vi "Raspberry Pi Compatible Compiler for LabVIEW.vi"() -> ()   [LabVIEW 2014, in "Raspberry Pi Compatible Compiler for LabVIEW.lvlib"]
uses:
  Raspberry Pi Compatible Compiler for LabVIEW.lvlib
  Custom Controls/CompileType.ctl
  RasPi_Services/Download/RuntimeVersion.ctl
  Custom Controls/Local Setup Parameters.ctl
  <vilib>/Platform/browser.llb/Open URL in Default Browser (string).vi
  RasPi_Services/Autodetect/Autodetect.lvlib
  RasPi_Services/Downloader/Downloader.lvclass
  Messaging/SimpleMessaging.lvlib
  RasPi_Services/Download/RasPiDownloader.lvlib
panel:
  in  "exit":bool
  in  "state variables":T2
  in  "Watermark":enum32{"Page 1", "Page 2"}(tab)
  in  "Compile Locally":bool
  out "Animated Image":i16(ring) caption="Ring 2"
  in  "Compilation Type":T3
  in  "Verify Connectivity":bool
  in  "Delete IP":bool
  in  "Edit IP":bool
  in  "Add Ip":bool
  in  "IP List":i32(listbox)
  in  "Blocker":string caption="Status"
  in  "Status":string
  out "Running":bool
  out "VIPath":path caption="Deploy .vi"
  out "StopStat":bool
  in  "FP":bool
  in  "Download":bool
  in  "Help":bool
  in  "Open":bool
  out "Busy":u16(ring)=12
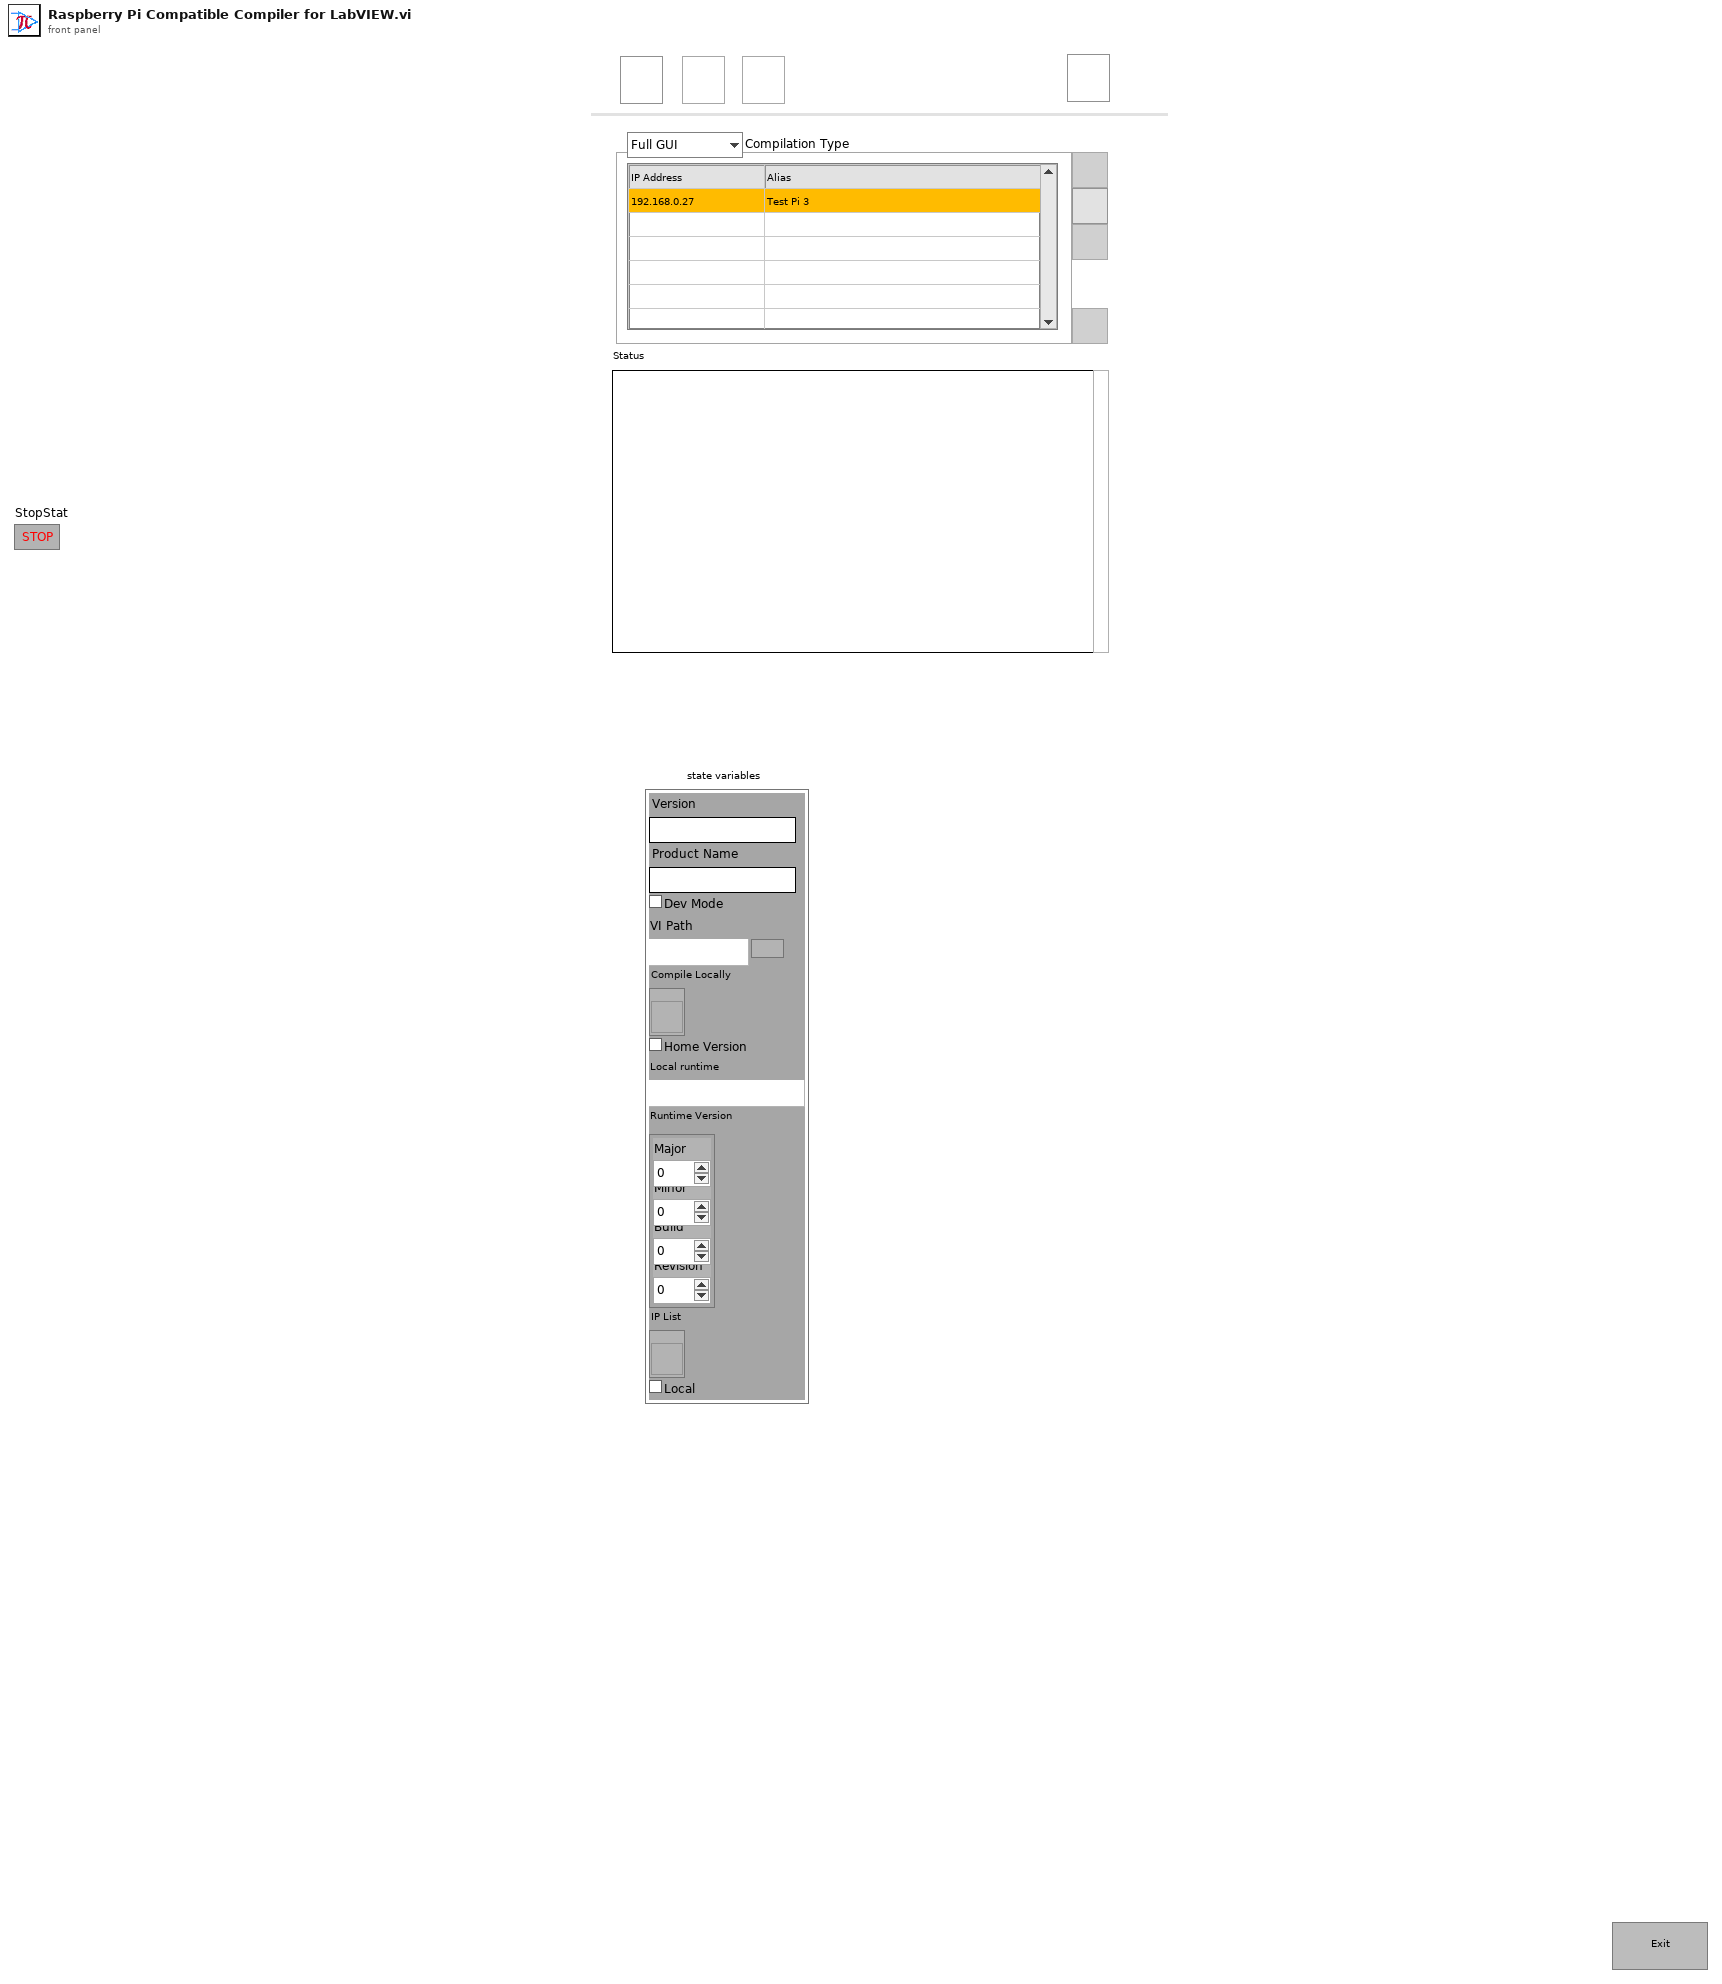
[diagram p1: front panel]
types:
  T1 = typedef "Raspberry Pi Compatible Compiler for LabVIEW.lvlib/RasPiDownloader.lvlib/RuntimeVersion.ctl" = cluster{"Major":i32, "Minor":i32, "Build":i32, "Revision":i32}
  T2 = cluster{"Version":string, "Product Name":string, "Dev Mode":bool, "VI Path":path, "Compile Locally":refnum<vi>, "Home Version":bool, "Local runtime":path, "Runtime Version":T1, "IP List":refnum<vi>, "Local":bool}
  T3 = typedef "Raspberry Pi Compatible Compiler for LabVIEW.lvlib/CompileType.ctl" = enum16{"Full GUI", "Console App"}
  T4 = typedef "Raspberry Pi Compatible Compiler for LabVIEW.lvlib/SimpleMessaging.lvlib/MessageQueueTD.ctl" = refnum<queue>
  T5 = enum8{"Enabled", "Disabled", "Disabled and Grayed Out"}
  T6 = typedef "Raspberry Pi Compatible Compiler for LabVIEW.lvlib/Local Setup Parameters.ctl" = enum16{"Add Last VI", "Read Last VI", "Add Board IP", "Remove Board IP", "Read All Board IP", "Add Runtime Version", "Read Runtime Version", "Add Package Version", "Read Package Version", "Add VIPCheck Time", "Read VIPCheck Time"}
  T7 = enum16{"Add IP", "Delete IP", "Get IP", "Edit IP"}
  T8 = typedef "Raspberry Pi Compatible Compiler for LabVIEW.lvlib/Autodetect.lvlib/UDP_Response_TD.ctl" = cluster{"IP address":string, "Port":u16, "response":string}
  T9 = typedef "Raspberry Pi Compatible Compiler for LabVIEW.lvlib/Autodetect.lvlib/UDP_HostinfoTD.ctl" = cluster{"hostname":string, "version":string}
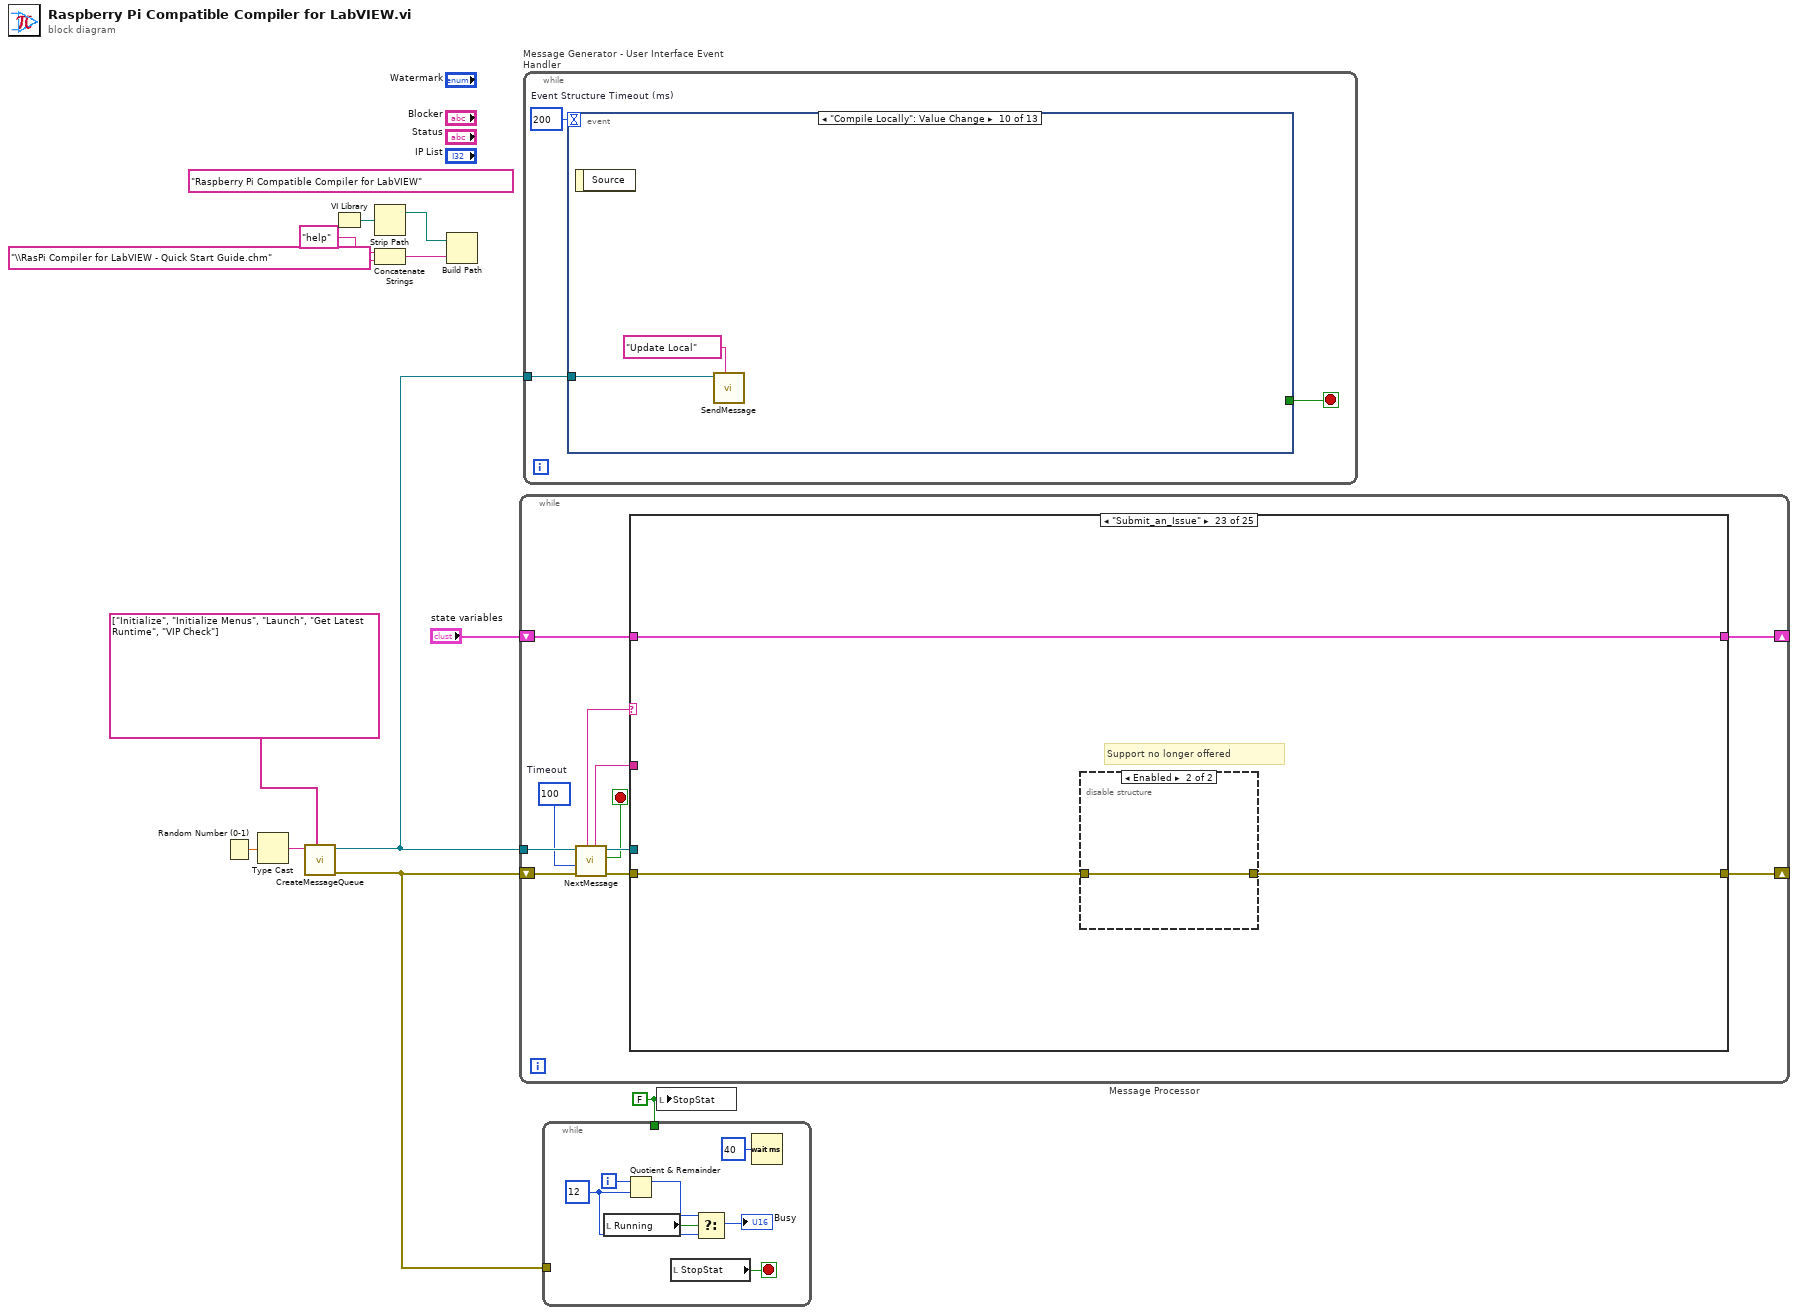
[diagram p0: block diagram]
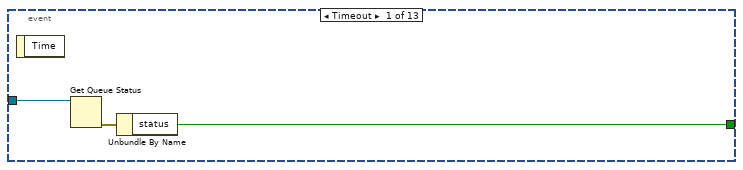
[diagram p2: hidden frame]
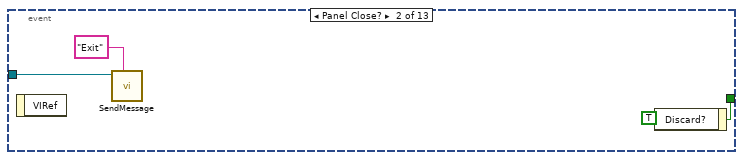
[diagram p3: hidden frame]
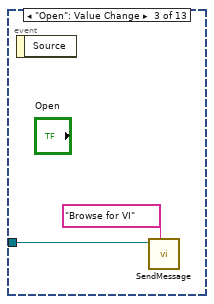
[diagram p4: hidden frame]
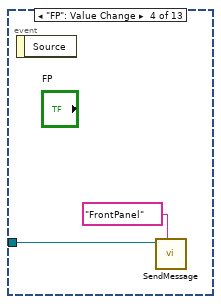
[diagram p5: hidden frame]
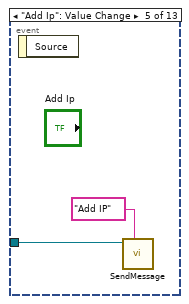
[diagram p6: hidden frame]
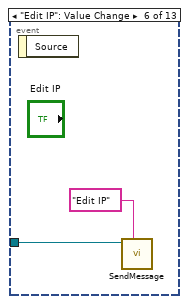
[diagram p7: hidden frame]
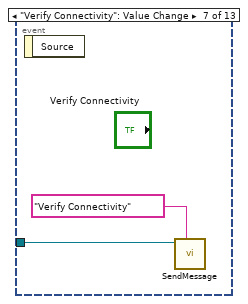
[diagram p8: hidden frame]
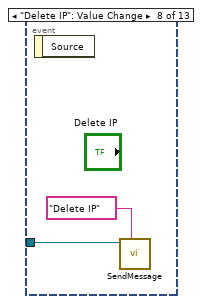
[diagram p9: hidden frame]
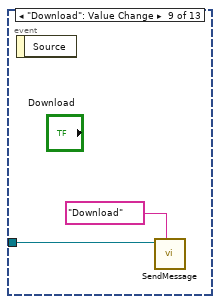
[diagram p10: hidden frame]
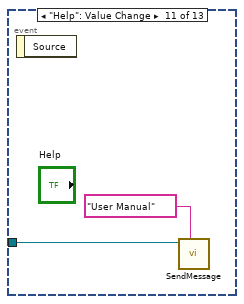
[diagram p11: hidden frame]
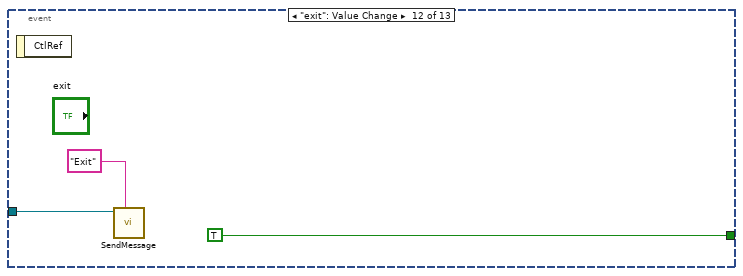
[diagram p12: hidden frame]
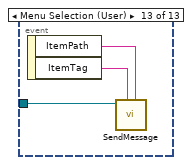
[diagram p13: hidden frame]
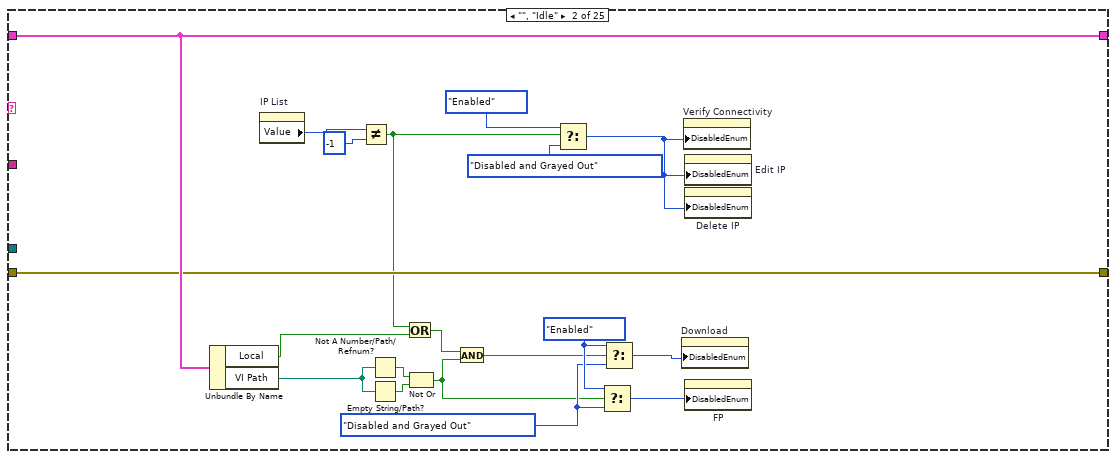
[diagram p15: hidden frame]
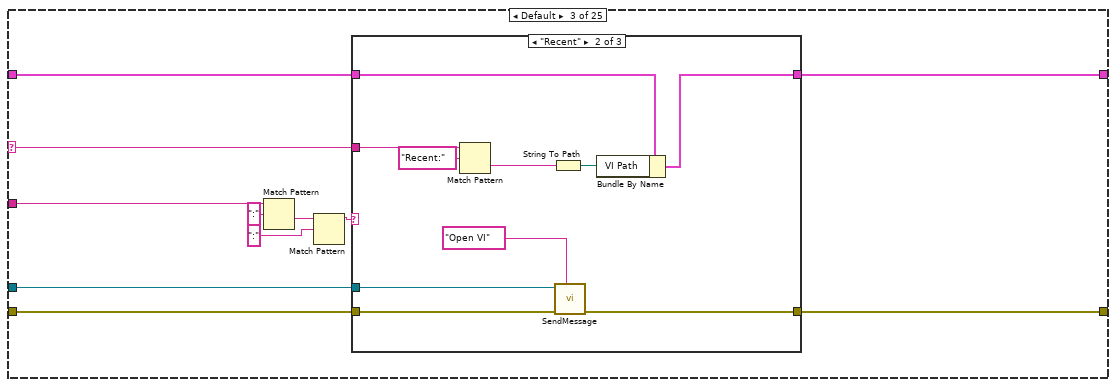
[diagram p16: hidden frame]
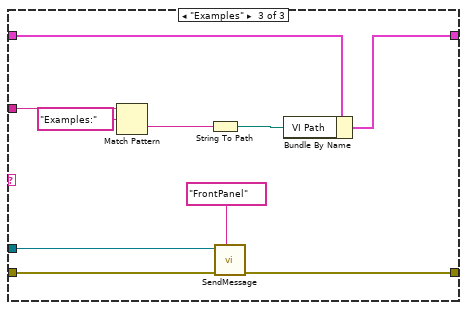
[diagram p18: hidden frame]
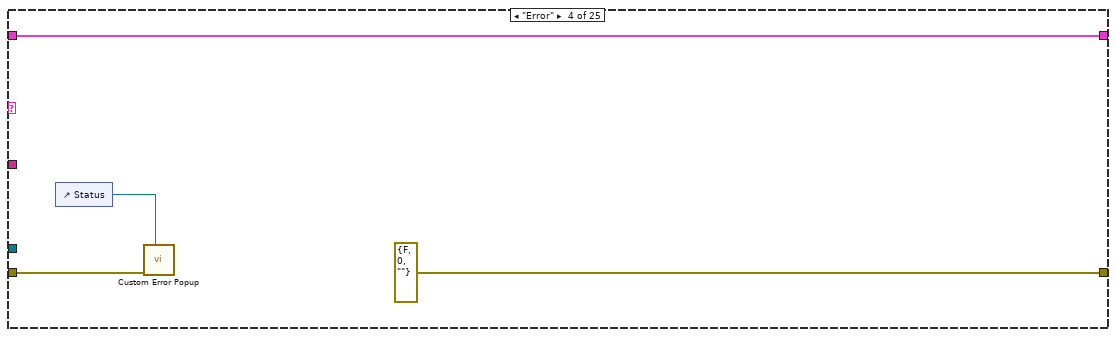
[diagram p19: hidden frame]
diagram:
  w7 = FALSE ("StopStat")
  (unwired) "Raspberry Pi Compatible Compiler for LabVIEW" ("menu tag")
  n1 = Random Number (0-1)() -> (number: 0 to 1=w2:dbl)
  n2 = Type Cast(x=w2) -> (*(type *) &x=w3:string)  [unwired: 1 in]
  n3 = call "CreateMessageQueue.vi"("initial message names"=string[] ["Initialize", "Initialize Menus", "Launch", "Get Latest Runtime", "VIP Check"], "message queue name"=w3) -> ("error out"=w1:errorcluster, "message queue out"=w5:T4)  [unwired: 5 in, 1 out]
  n4 = VI Library() -> (path=w10:path)
  n5 = Strip Path(path=w10) -> (stripped path=w11:path)  [unwired: 1 out]
  n6 = Concatenate Strings("help" ("name or relative path"), "\\RasPi Compiler for LabVIEW - Quick Start Guide.chm" ("name or relative path")) -> (w9:string)
  n7 = Build Path(base path=w11, name or relative path=w9) -> ()  [unwired: 1 out]
  n8 = while "Message Processor" {
    shift-left: w1 -> [w18]
    shift-right: [w21] -> _
    tunnel: w5 -> [w19]
    shift-left: "state variables" -> [w23]
    shift-right: [w22] -> _
    stop <- w13 stop-if-true
    w16 = 100  # Timeout
    n9 = call "NextMessage.vi"("error in"=w18, "timeout in ms (-1)"=w16, "message queue in"=w19) -> ("error out"=w17:errorcluster, "exit"=w13:bool, "message queue out"=w20:T4, "Value"=w14:string, "Name"=w15:string)  [unwired: 1 in, 1 out]
    n10 = case shown="\"Submit_an_Issue\"" w15 {
      selector: w15 -> [_ _ w51 _ _ _ _ _ _ _ _ _ _ _ _ _ _ _ _ _ _ _ _ _ _]
      tunnel: [w25 w35 w46 w81 w83 w111 w123 w140 w188 w224 w238 w246 w248 w249 w284 w317 w330 w335 w348 w368 w403 w415 w418 w428 w433] -> w22
      tunnel: w23 -> [w25 w35 w47 w81 w83 w113 w123 w141 w189 w226 w239 w246 w248 w250 w284 w317 w330 w335 w348 w368 w403 w415 w418 w428 w436]
      tunnel: w20 -> [_ _ w48 _ _ _ _ _ w182 _ _ w244 _ w251 _ _ _ _ _ _ _ _ _ w425 _]
      tunnel: w17 -> [w24 w34 w50 w79 w82 w94 w126 w143 w191 w228 w237 w245 w247 w253 w287 w318 w333 w337 w351 w370 w407 w413 w417 w427 w437]
      tunnel: [w24 w34 w49 errorcluster {"status"=FALSE, "code"=0, "source"=""} ("error out") w82 w87 w125 _ w181 w221 w237 w240 w247 w252 w286 w319 w332 w336 w349 w369 w405 w412 w416 w426 w430] -> w21
      tunnel: w14 -> [_ _ w45 _ _ _ _ _ w177 _ _ _ _ _ _ _ _ _ _ _ _ _ _ _ _]
      frame "---------- Framework Operations ----------" {
      }
      frame "", "Idle" {
        w33 = T5."Disabled and Grayed Out" ("Disabled")
        w38 = T5."Enabled" ("Disabled")
        n11 = Unbundle By Name(w35) -> ("Local"=w26:bool, "VI Path"=w30:path)
        n12 = property on="IP List" class="MCListbox (strict)"() -> ("Value"=w44:i32)  [unwired: 2 in, 2 out]
        n13 = Not Equal?(x=w44, y=-1) -> (x != y?=w31:bool)
        n14 = Not A Number/Path/Refnum?(number/path/refnum=w30) -> (NaN/Path/Refnum?=w28:bool)
        n15 = Empty String/Path?(string/path=w30) -> (empty?=w29:bool)
        n16 = Or(x=w31, y=w26) -> (x .or. y?=w32:bool)
        n17 = Not Or(1:w29, 2:w28) -> (0:w27:bool)
        n18 = And(x=w32, y=w27) -> (x .and. y?=w36:bool)
        n19 = Select(t=T5."Enabled", s=w31, f=T5."Disabled and Grayed Out" ("Disabled")) -> (s? t:f=w40:T5)
        n20 = Select(t=w38, s=w27, f=w33) -> (s? t:f=w37:T5)
        n21 = Select(t=w38, s=w36, f=w33) -> (s? t:f=w39:T5)
        n22 = property on="Download" class="Bool"("DisabledEnum"=w39) -> ()  [unwired: 2 in, 2 out]
        n23 = property on="Verify Connectivity" class="Bool"("DisabledEnum"=w40) -> ()  [unwired: 2 in, 2 out]
        n24 = property on="Edit IP" class="Bool"("DisabledEnum"=w40) -> ()  [unwired: 2 in, 2 out]
        n25 = property on="Delete IP" class="Bool"("DisabledEnum"=w40) -> ()  [unwired: 2 in, 2 out]
        n26 = property on="FP" class="Bool"("DisabledEnum"=w37) -> ()  [unwired: 2 in, 2 out]
      }
      frame Default {
        n27 = Match Pattern(string=w45, regular expression=":") -> (after substring=w53:string)  [unwired: 1 in, 3 out]
        n28 = Match Pattern(string=w53, regular expression=":") -> (before substring=w55:string)  [unwired: 1 in, 3 out]
        n29 = case shown="\"Recent\"" w55 {
          tunnel: w51 -> [_ w66 w76]
          tunnel: w50 -> [w57 w63 w72]
          tunnel: w48 -> [_ w64 w71]
          tunnel: [w57 w62 w73] -> w49
          tunnel: w47 -> [w56 w60 w70]
          tunnel: [w56 w58 w68] -> w46
          frame Default {
          }
          frame "Recent" {
            n30 = Match Pattern(string=w66, regular expression="Recent:") -> (after substring=w65:string)  [unwired: 1 in, 3 out]
            n31 = String To Path(string=w65) -> (path=w59:path)
            n32 = call "SendMessage.vi"("Name"="Open VI" ("Command"), "error in"=w63, "message queue in"=w64) -> ("error out"=w62:errorcluster)  [unwired: 4 in, 2 out]
            n33 = Bundle By Name(cluster=w60, "VI Path"=w59) -> (w58:T2)
          }
          frame "Examples" {
            n34 = Match Pattern(string=w76, regular expression="Examples:") -> (after substring=w75:string)  [unwired: 1 in, 3 out]
            n35 = String To Path(string=w75) -> (path=w69:path)
            n36 = call "SendMessage.vi"("Name"="FrontPanel", "error in"=w72, "message queue in"=w71) -> ("error out"=w73:errorcluster)  [unwired: 4 in, 2 out]
            n37 = Bundle By Name(cluster=w70, "VI Path"=w69) -> (w68:T2)
          }
        }
      }
      frame "Error" {
        n38 = control-ref of="Status"() -> (w78:refnum<vi>)
        n39 = call "Custom Error Popup.vi"("Message Box"=w78, "error in (no error)"=w79) -> ()  [unwired: 9 in, 1 out]
      }
      frame "---------- Generic Operations ----------" {
      }
      frame "Initialize" {
        w91 = FALSE ("Visible")
        n40 = control-ref of="Compile Locally"() -> (w93:refnum<vi>)
        n41 = property on="Watermark" class="TabCtl (strict)"(error in=w94, "Value"=enum32{"Page 1", "Page 2"}."Page 2" ("Watermark")) -> (error out=w100:errorcluster)  [unwired: 1 in, 1 out]
        n42 = property class="Bool (strict)"(reference=w93, error in=w100, "Visible"=w91, "Value"=w91) -> (reference out=w101:refnum<vi>, error out=w89:errorcluster)
        n43 = property on="FP" class="Bool"("DisabledEnum"=T5."Disabled and Grayed Out" ("Disabled")) -> ()  [unwired: 2 in, 2 out]
        n44 = Current VI's Menubar() -> (w102:refnum<k9>)
        n45 = Enable Menu Tracking(2:w89, 3:FALSE ("enable (T)"), 4:w102) -> (0:w88:errorcluster)  [unwired: 1 out]
        n46 = property on="IP List" class="MCListbox (strict)"("Value"=-1 ("IP List"), "ItemNames"=string[][] [] ("Item Names")) -> ()  [unwired: 2 in, 2 out]
        n47 = case shown="True" FALSE {
          tunnel: w101 -> [_ w122]
          tunnel: w88 -> [w114 w120]
          tunnel: [w114 w119] -> w87
          tunnel: [FALSE ("Student") w118] -> w86
          tunnel: [TRUE ("Dev Machine") w117] -> w85
          frame False {
          }
          frame True {
            n48 = Current VI's Path() -> (path=w121:path)
            n49 = call "DevMode.vi"("error in (no error)"=w120, "Compile Locally"=w122, "path"=w121) -> ("error out"=w119:errorcluster, "Student"=w118:bool, "Dev Machine"=w117:bool)  [unwired: 6 in]
          }
        }
        n50 = Select(t=enum32{"Page 1", "Page 2"}."Page 1" ("Watermark"), s=w86, f=enum32{"Page 1", "Page 2"}."Page 2") -> (s? t:f=w97:enum32{"Page 1", "Page 2"})
        n51 = property on="Watermark" class="TabCtl (strict)"("Value"=w97) -> ()  [unwired: 2 in, 2 out]
        n52 = property on="Busy" class="Ring (strict)"("Value"=u16 12 ("Busy"), "Visible"=FALSE) -> ()  [unwired: 2 in, 2 out]
        n53 = control-ref of="IP List"() -> (w92:refnum<vi>)
        n54 = local write "StopStat"(FALSE ("StopStat")) -> ()
        n55 = local write "Status"("") -> ()
        n56 = Bundle By Name(cluster=w113, "Product Name"="Raspberry Pi Compatible Compiler for LabVIEW" ("menu tag"), "VI Path"=path "" ("VIPath"), "Compile Locally"=w93, "Dev Mode"=w85, "Home Version"=w86, "IP List"=w92) -> (w111:T2)
        "Running" <- FALSE ("Running")
      }
      frame "Initialize Menus" {
        n57 = Current VI's Menubar() -> (w139:refnum<k9>)
        n58 = call "Local Setup Config.vi"("Local Setup Param"=Local_Setup_Parameters."Read Last VI", "error in"=w126) -> ("LastVIs"=w129:string[], "error out"=w128:errorcluster)  [unwired: 10 in, 2 out]
        n59 = Unbundle By Name(w123) -> ("Product Name"=w124:string)
        n60 = call "Update Last VI List to Menu.vi"("LastVIs"=w129, "menu reference"=w139, "error in (no error)"=w128) -> ("error out"=w130:errorcluster)  [unwired: 12 in]
        n61 = call "Local Setup Config.vi"("Local Setup Param"=Local_Setup_Parameters."Read All Board IP", "error in"=w130) -> ("KeyValues"=w133:string[], "KeyNames"=w132:string[], "error out"=w136:errorcluster)  [unwired: 10 in, 1 out]
        n62 = Build Array(w132, w133) -> (w134:string[][])
        n63 = call "Load Examples.vi"("menu reference"=w139, "error in (no error)"=w136, "Release Name"=w124) -> ("error out"=w138:errorcluster)  [unwired: 8 in]
        n64 = Transpose 2D Array(2D array=w134) -> (transposed array=w135:string[][])
        n65 = property on="IP List" class="MCListbox (strict)"("ItemNames"=w135) -> ()  [unwired: 2 in, 2 out]
        n66 = Enable Menu Tracking(2:w138, 3:TRUE ("enable (T)"), 4:w139) -> (0:w125:errorcluster)  [unwired: 1 out]
      }
      frame "Launch" {
        n67 = property class="App"(error in=w143) -> (reference out=w155:refnum<vi>, error out=w156:errorcluster, "App.MenuLaunchVI"=w153:string, "App.MenuLaunchApp"=w154:refnum<vi>)  [unwired: 1 in]
        n68 = Close Reference(reference=w155, error in (no error)=w156) -> (error out=w157:errorcluster)
        n69 = Unbundle By Name(w141) -> ("Product Name"=w142:string)
        n70 = Open VI Reference(application reference (local)=w154, vi path=w153, error in (no error)=w157) -> (vi reference=w150:refnum<vi>, error out=w149:errorcluster)  [unwired: 3 in]
        n71 = property class="VI"(reference=w150, error in=w149) -> (reference out=w152:refnum<vi>, error out=w151:errorcluster, "Path"=w159:path)
        n72 = Close Reference(reference=w152, error in (no error)=w151) -> (error out=w148:errorcluster)
        n73 = Strip Path(path=w159) -> (name=w162:string)  [unwired: 1 out]
        n74 = Empty String/Path?(string/path=w162) -> (empty?=w146:bool)
        n75 = Not Equal?(x=w162, y="GettingStartedWindow.vi") -> (x != y?=w144:bool)
        n76 = Unbundle By Name(w148) -> ("status"=w147:bool)
        n77 = call <vilib>:"Clear Errors.vi"("error in (no error)"=w148) -> ()  [unwired: 5 in, 2 out]
        n78 = Compound Arithmetic op=AND(invert w147, invert w146, w144) -> (w158:bool)
        n79 = case shown="True" w158 {
          tunnel: w159 -> [_ w167]
          tunnel: w142 -> [w165 w172]
          tunnel: w162 -> [_ w171]
          tunnel: [w165 w170] -> w160
          tunnel: [T5."Disabled and Grayed Out" ("Disabled") T5."Enabled" ("Disabled")] -> w161
          tunnel: w141 -> [w163 w168]
          tunnel: [w163 w166] -> w140
          frame False {
          }
          frame True {
            n80 = Bundle By Name(cluster=w168, "VI Path"=w167) -> (w166:T2)
            n81 = Concatenate Strings(w172, " - " ("string"), w171) -> (w170:string)
          }
        }
        n82 = property on="FP" class="Bool"("DisabledEnum"=w161) -> ()  [unwired: 2 in, 2 out]
        n83 = property on="Download" class="Bool"("DisabledEnum"=w161) -> ()  [unwired: 2 in, 2 out]
        n84 = property class="VI"("Front Panel.Title"=w160) -> ()  [unwired: 2 in, 2 out]
      }
      frame "VIP Check" {
        n85 = Scan From String(input string=w177, default 1=FALSE ("Force Check(F)")) -> (error out=w174:errorcluster, output 1=w175:bool)  [unwired: 3 in, 2 out]
        n86 = call <vilib>:"Clear Errors.vi"("error in (no error)"=w174) -> ()  [unwired: 5 in, 2 out]
        n87 = Unbundle By Name(w189) -> ("Product Name"=w190:string, "Home Version"=w187:bool, "Dev Mode"=w178:bool)
        n88 = call "VIP Check.vi"("Dev Mode"=w178, "Force Check(F)"=w175, "error in"=w191, "Home version"=w187, "Product Name"=w190) -> ("error out"=w180:errorcluster, "available version"=w184:string, "Update available"=w185:bool, "Continue"=w186:bool, "Check Version"=w179:bool, "current version"=w183:string)  [unwired: 1 in]
        n89 = case shown="No Error" w180 {
          selector: w180 -> [w193 w220]
          tunnel: w186 -> [w199 _]
          tunnel: w185 -> [w198 _]
          tunnel: w184 -> [w197 _]
          tunnel: w183 -> [w196 w216]
          tunnel: w182 -> [w195 _]
          tunnel: [w194 w215] -> w181
          tunnel: w179 -> [w192 _]
          frame No Error {
            n90 = case shown="False" w199 {
              tunnel: w198 -> [_ _]
              tunnel: w197 -> [_ w212]
              tunnel: w196 -> [_ w211]
              tunnel: w195 -> [w203 _]
              tunnel: w193 -> [w202 w214]
              tunnel: [w201 w214] -> w194
              tunnel: w192 -> [w200 _]
              frame False {
                n91 = case shown="True" w200 {
                  tunnel: w203 -> [_ w207]
                  tunnel: w202 -> [w204 w206]
                  tunnel: [w204 w205] -> w201
                  frame False {
                  }
                  frame True {
                    n92 = call "SendMessage.vi"("Name"="Exit", "error in"=w206, "message queue in"=w207) -> ("error out"=w205:errorcluster)  [unwired: 4 in, 2 out]
                  }
                }
              }
              frame True {
                n93 = local read "Status"() -> (w210:string)
                n94 = Format Into String(format string="A different version is available:\nInstalled : %s\nReleased : %s\n\nNavigate to the Compiler Menu and select Compiler-> Check for Updates to upgrade", initial string=w210, w211, w212) -> (resulting string=w213:string)  [unwired: 1 in, 1 out]
                n95 = local write "Status"(w213) -> ()
              }
            }
          }
          frame Error {
            n96 = call <vilib>:"Clear Errors.vi"("error in (no error)"=w220) -> ("error out"=w215:errorcluster)  [unwired: 5 in, 1 out]
            n97 = local read "Status"() -> (w218:string)
            n98 = Format Into String(format string="Compiler Version Installed : %s\n\nVersion Update Check Couldn't Be Performed as Dev Machine Couldn't Connect to Public Repository", initial string=w218, w216) -> (resulting string=w219:string)  [unwired: 1 in, 1 out]
            n99 = local write "Status"(w219) -> ()
          }
        }
        n100 = Bundle By Name(cluster=w189, "Version"=w183) -> (w188:T2)
      }
      frame "Get Latest Runtime" {
        n101 = call "Runtime Version.vi"("error in"=w228) -> ("error out"=w223:errorcluster, "Runtime Version"=w222:string, "Version"=w227:T1, "Local runtime"=w225:path)  [unwired: 5 in]
        n102 = Bundle By Name(cluster=w226, "Local runtime"=w225, "Runtime Version"=w227) -> (w224:T2)
        n103 = case shown="Error" w223 {
          selector: w223 -> [w229 w235]
          tunnel: w222 -> [_ w231]
          tunnel: [w229 w230] -> w221
          frame No Error {
          }
          frame Error {
            n104 = call <vilib>:"Clear Errors.vi"("error in (no error)"=w235) -> ("error out"=w230:errorcluster)  [unwired: 5 in, 1 out]
            n105 = local read "Status"() -> (w233:string)
            n106 = Format Into String(format string="Runtime Version Installed : %s\n\nVersion Update Check Couldn't Be Performed as Dev Machine Couldn't Connect to Public Repository", initial string=w233, w231) -> (resulting string=w234:string)  [unwired: 1 in, 1 out]
            n107 = local write "Status"(w234) -> ()
          }
        }
      }
      frame "Update Local" {
        n108 = Bundle By Name(cluster=w239, "Local"="Compile Locally") -> (w238:T2)
      }
      frame "Exit" {
        n109 = Release Queue(queue=w244, error in (no error)=w245) -> (error out=w241:errorcluster)  [unwired: 1 in, 2 out]
        n110 = Current VI's Path() -> (path=w243:path)
        n111 = call "Close VI FP.vi"("error in (no error)"=w241, "path"=w243) -> ("error out"=w240:errorcluster)  [unwired: 9 in]
        "StopStat" <- TRUE ("StopStat")
      }
      frame "---------- Application Operations ----------" {
      }
      frame "Browse for VI", "Open" {
        n112 = call "File Dialog2"("error in"=w253, "pattern (all files)"="*.vi") -> ("selected path"=w254:path, "exists"=w255:bool, "error out"=w256:errorcluster)  [unwired: 10 in, 1 out]
        n113 = case shown="True" w255 {
          tunnel: w256 -> [w260 w267]
          tunnel: w254 -> [_ w266]
          tunnel: [w259 w268] -> w252
          tunnel: w251 -> [_ w264]
          tunnel: w250 -> [w258 w262]
          tunnel: [w258 w261] -> w249
          frame False {
            n114 = call <vilib>:"Clear Errors.vi"("error in (no error)"=w260) -> ("error out"=w259:errorcluster)  [unwired: 5 in, 1 out]
          }
          frame True {
            n115 = call "Is VI Runnable.vi"("error in (no error)"=w267, "selected path"=w266) -> ("error out"=w265:errorcluster)  [unwired: 9 in]
            n116 = case shown="No Error" w265 {
              selector: w265 -> [w271 w281]
              tunnel: [w272 w281] -> w268
              tunnel: w266 -> [w274 w280]
              tunnel: w264 -> [w270 _]
              tunnel: [_ w277] -> w263
              tunnel: w262 -> [w275 w276]
              tunnel: [w273 w276] -> w261
              frame No Error {
                n117 = Bundle By Name(cluster=w275, "VI Path"=w274) -> (w273:T2)
                n118 = call "SendMessage.vi"("Name"="Open VI" ("Command"), "error in"=w271, "message queue in"=w270) -> ("error out"=w272:errorcluster)  [unwired: 4 in, 2 out]
              }
              frame Error {
                n119 = Path To String(path=w280) -> (string=w279:string)
                n120 = Format Into String(initial string="Error VI is not runnable\nPath: " ("pattern (all files)"), w279) -> (resulting string=w277:string)  [unwired: 2 in, 1 out]
              }
            }
            n121 = local write "Status"(w263) -> ()
          }
        }
      }
      frame "Open VI" {
        n122 = Unbundle By Name(w284) -> ("Product Name"=w282:string, "VI Path"=w285:path)
        n123 = Current VI's Menubar() -> (w283:refnum<k9>)
        n124 = call "Is VI Runnable.vi"("error in (no error)"=w287, "selected path"=w285) -> ("error out"=w288:errorcluster)  [unwired: 9 in]
        n125 = case shown="No Error" w288 {
          selector: w288 -> [w298 w315]
          tunnel: w282 -> [w308 _]
          tunnel: w283 -> [w295 _]
          tunnel: [w293 w315] -> w286
          tunnel: w285 -> [w303 w314]
          tunnel: [w302 w313] -> w289
          tunnel: ["Loaded: " ("pattern (all files)") "Error Loading: " ("pattern (all files)")] -> w290
          tunnel: [T5."Enabled" ("Disabled") T5."Disabled and Grayed Out" ("Disabled")] -> w292
          frame No Error {
            n126 = Strip Path(path=w303) -> (name=w307:string)  [unwired: 1 out]
            n127 = Path To String(path=w303) -> (string=w302:string)
            n128 = Concatenate Strings(w308, " - " ("string"), w307) -> (w309:string)
            n129 = property class="VI"("Front Panel.Title"=w309) -> ()  [unwired: 2 in, 2 out]
            n130 = Enable Menu Tracking(2:w298, 3:FALSE ("enable (T)"), 4:w295) -> (0:w297:errorcluster)  [unwired: 1 out]
            n131 = call "Local Setup Config.vi"("Local Setup Param"=Local_Setup_Parameters."Add Last VI", "Last VI"=w302, "error in"=w297) -> ("LastVIs"=w304:string[], "error out"=w305:errorcluster)  [unwired: 9 in, 2 out]
            n132 = call "Update Last VI List to Menu.vi"("LastVIs"=w304, "menu reference"=w295, "error in (no error)"=w305) -> ("error out"=w294:errorcluster)  [unwired: 12 in]
            n133 = Enable Menu Tracking(2:w294, 3:TRUE ("enable (T)"), 4:w295) -> (0:w293:errorcluster)  [unwired: 1 out]
          }
          frame Error {
            n134 = Path To String(path=w314) -> (string=w313:string)
          }
        }
        n135 = Format Into String(initial string=w290, w289) -> (resulting string=w291:string)  [unwired: 2 in, 1 out]
        n136 = property on="Download" class="Bool"("DisabledEnum"=w292) -> ()  [unwired: 2 in, 2 out]
        n137 = local write "Status"(w291) -> ()
      }
      frame "FrontPanel" {
        n138 = Unbundle By Name(w317) -> ("VI Path"=w316:path)
        n139 = call "Open VI FP.vi"("error in (no error)"=w318, "VIPath"=w316) -> ("error out"=w320:errorcluster)  [unwired: 9 in]
        n140 = case shown="No Error" w320 {
          selector: w320 -> [w321 _]
          tunnel: [w321 _] -> w319
          tunnel: w316 -> [_ w325]
          frame No Error {
          }
          frame Error {
            n141 = Empty String/Path?(string/path=w325) -> (empty?=w329:bool)
            n142 = Not A Number/Path/Refnum?(number/path/refnum=w325) -> (NaN/Path/Refnum?=w328:bool)
            n143 = Or(x=w328, y=w329) -> (x .or. y?=w327:bool)
            n144 = Format Into String(initial string="Error opening Front Panel\nPath: " ("false string"), w325) -> (resulting string=w323:string)  [unwired: 2 in, 1 out]
            n145 = Append True/False String(1:w327, 2:w323, 3:"No VI loaded" ("true string")) -> (0:w322:string)  [unwired: 1 in]
            n146 = local write "Status"(w322) -> ()
          }
        }
      }
      frame "About" {
        n147 = Unbundle By Name(w330) -> ("Version"=w331:string)
        n148 = call "About Dialog.vi"("error in (no error)"=w333, "SW Version"=w331) -> ("error out"=w332:errorcluster)  [unwired: 9 in]
      }
      frame "Add IP" {
        w341 = "" ("IP Address")
        n149 = Unbundle By Name(w335) -> ("IP List"=w334:refnum<vi>)
        n150 = call "Add IP Address.vi"("error in"=w337, "Alias"=w341, "IP Address"=w341) -> ("error out"=w338:errorcluster, "Alias to Add"=w340:string, "IP to Add"=w339:string)  [unwired: 6 in]
        n151 = call "Edit List.vi"("Method"=enum16{"Add IP", "Delete IP", "Get IP"}."Add IP", "error in (no error)"=w338, "Alias"=w340, "IP Address"=w339, "IP List"=w334) -> ("error out"=w343:errorcluster, "Alias"=w346:string, "IP Address"=w345:string)  [unwired: 3 in, 1 out]
        n152 = call "Local Setup Config.vi"("KeyName"=w345, "Local Setup Param"=Local_Setup_Parameters."Add Board IP", "KeyValue"=w346, "error in"=w343) -> ("error out"=w336:errorcluster)  [unwired: 8 in, 3 out]
      }
      frame "Edit IP" {
        n153 = Unbundle By Name(w348) -> ("IP List"=w347:refnum<vi>)
        n154 = call "Edit List.vi"("Method"=enum16{"Add IP", "Delete IP", "Get IP"}."Get IP", "error in (no error)"=w351, "IP List"=w347) -> ("error out"=w364:errorcluster, "Alias"=w355:string, "IP Address"=w356:string, "Selected Line"=w350:i32)  [unwired: 5 in]
        n155 = call "Add IP Address.vi"("Connected(F)"=TRUE, "error in"=w364, "Alias"=w355, "IP Address"=w356) -> ("error out"=w363:errorcluster, "Alias to Add"=w362:string, "IP to Add"=w361:string)  [unwired: 5 in]
        n156 = call "Edit List.vi"("Selected Line"=w350, "Method"=T7."Edit IP", "error in (no error)"=w363, "Alias"=w362, "IP Address"=w361, "IP List"=w347) -> ("error out"=w365:errorcluster, "Alias"=w353:string, "IP Address"=w354:string)  [unwired: 2 in, 1 out]
        n157 = call "Local Setup Config.vi"("KeyName"=w356, "Local Setup Param"=Local_Setup_Parameters."Remove Board IP", "KeyValue"=w355, "error in"=w365) -> ("error out"=w358:errorcluster)  [unwired: 8 in, 3 out]
        n158 = call "Local Setup Config.vi"("KeyName"=w354, "Local Setup Param"=Local_Setup_Parameters."Add Board IP", "KeyValue"=w353, "error in"=w358) -> ("error out"=w349:errorcluster)  [unwired: 8 in, 3 out]
      }
      frame "Verify Connectivity" {
        n159 = Unbundle By Name(w368) -> ("IP List"=w367:refnum<vi>)
        n160 = call "Edit List.vi"("Method"=enum16{"Add IP", "Delete IP", "Get IP"}."Get IP", "error in (no error)"=w370, "IP List"=w367) -> ("error out"=w379:errorcluster, "IP Address"=w372:string)  [unwired: 5 in, 2 out]
        n161 = local write "Status"("connecting" ("Status")) -> ()
        n162 = Unbundle By Name(w379) -> ("status"=w378:bool)
        n163 = call "Unicast_UDP_message.vi"("message"="*IDN?", "error in"=w379, "address"=w372) -> ("error out"=w374:errorcluster, "response"=w375:T8)  [unwired: 5 in]
        n164 = Not(x=w378) -> (.not. x?=w380:bool)
        n165 = case shown="No Error" w374 {
          selector: w374 -> [w392 w401]
          tunnel: [w385 w402] -> w369
          tunnel: w375 -> [w394 _]
          tunnel: "Connection Couldn't Be Established" ("response") -> [w397 w400]
          tunnel: [w396 w400] -> w383
          tunnel: [FALSE ("Boolean") _] -> w382
          frame No Error {
            n166 = call "ParseHostInfo.vi"("error in"=w392, "response"=w394) -> ("error out"=w391:errorcluster, "Cluster"=w393:cluster{"IP address":string, "host info":T9})  [unwired: 8 in]
            n167 = Unbundle By Name(w393) -> ("host info.hostname"=w390:string, "host info.version"=w387:string)
            n168 = call <vilib>:"Clear Errors.vi"("error in (no error)"=w391) -> ("error out"=w385:errorcluster)  [unwired: 5 in, 1 out]
            n169 = Format Into String(format string="Hostname: %s\nRuntime Version: %s", initial string="Connection Successful\n" ("response"), w390, w387) -> (resulting string=w388:string)  [unwired: 1 in, 1 out]
            n170 = Not Equal?(x=w387, y="") -> (x != y?=w398:bool)
            n171 = Select(t=w388, s=w398, f=w397) -> (s? t:f=w396:string)
          }
          frame Error {
            n172 = call <vilib>:"Clear Errors.vi"("error in (no error)"=w401) -> ("error out"=w402:errorcluster)  [unwired: 5 in, 1 out]
          }
        }
        n173 = Boolean To (0,1)(Boolean=w380) -> (0, 1=→"Animated Image":i16)
        n174 = Boolean To (0,1)(Boolean=w382) -> (0, 1=w381:i16)
        n175 = local write "Animated Image"(w381) -> ()
        n176 = local write "Status"(w383) -> ()
      }
      frame "Delete IP" {
        n177 = Unbundle By Name(w403) -> ("IP List"=w404:refnum<vi>)
        n178 = call "Edit List.vi"("Method"=enum16{"Add IP", "Delete IP", "Get IP"}."Delete IP", "error in (no error)"=w407, "IP List"=w404) -> ("error out"=w406:errorcluster, "Alias"=w411:string, "IP Address"=w410:string)  [unwired: 5 in, 1 out]
        n179 = call "Local Setup Config.vi"("KeyName"=w410, "Local Setup Param"=Local_Setup_Parameters."Remove Board IP", "KeyValue"=w411, "error in"=w406) -> ("error out"=w405:errorcluster)  [unwired: 8 in, 3 out]
      }
      frame "QuickStart", "User Manual" {
        n180 = call-poly <vilib>:"Open URL in Default Browser.vi"("error in (no error)"=w413, "URL"="https://github.com/labviewforRaspi/LabVIEWforRasPi/wiki") -> ("error out"=w412:errorcluster)  [unwired: 4 in, 1 out]
      }
      frame "Submit_an_Issue" {
        # "Support no longer offered"
        n181 = disable-structure shown="Enabled" {
          disable-tunnel: w417 -> [w420 w421]
          disable-tunnel: [w419 w421] -> w416
          frame Disabled {
            n182 = call "Rasbperry Pi Compiler for LabVIEW Beta - Submit an Issue.vi"("error in (no error)"=w420) -> ("error out"=w419:errorcluster)  [unwired: 10 in]
          }
          frame Enabled {
          }
        }
      }
      frame "check_update" {
        n183 = Format Into String(TRUE) -> (resulting string=w422:string)  [unwired: 3 in, 1 out]
        n184 = call "SendMessage.vi"("Value"=w422, "Name"="VIP Check", "error in"=w427, "message queue in"=w425) -> ("error out"=w426:errorcluster)  [unwired: 3 in, 2 out]
      }
      frame "Download" {
        n185 = flat-sequence {
          tunnel: w436 -> [w442]
          tunnel: w437 -> [w445]
          tunnel: [w444] -> w435
          tunnel: [w442] -> w434
          tunnel: [w443] -> w431
          tunnel: w435 -> [w461]
          tunnel: w434 -> [w454]
          tunnel: [w454] -> w432
          tunnel: w431 -> [w453]
          tunnel: [w448] -> w429
          tunnel: [w482] -> w433
          tunnel: w432 -> [w482]
          tunnel: [w478] -> w430
          tunnel: w429 -> [w478]
          frame #0 {
            w440 = TRUE ("Running")
            n186 = Boolean To (0,1)(Boolean=w440) -> (0, 1=w439:i16)
            n187 = Unbundle By Name(w442) -> ("IP List"=w441:refnum<vi>)
            n188 = local write "Animated Image"(w439) -> ()
            n189 = local write "Running"(w440) -> ()
            n190 = local write "Status"("" ("Status")) -> ()
            n191 = property on="Busy" class="Ring (strict)"("Visible"=TRUE) -> ()  [unwired: 2 in, 2 out]
            n192 = call "Edit List.vi"("Method"=enum16{"Add IP", "Delete IP", "Get IP"}."Get IP", "error in (no error)"=w445, "IP List"=w441) -> ("error out"=w444:errorcluster, "IP Address"=w443:string)  [unwired: 5 in, 2 out]
          }
          frame #1 {
            n193 = Unbundle By Name(w454) -> ("Runtime Version"=w456:T1, "Local runtime"=w455:path)
            n194 = Unbundle By Name(w454) -> ("Local"=w459:bool, "VI Path"=w460:path)
            n195 = Current VI's Path() -> (path=w463:path)
            n196 = Strip Path(path=w463) -> (stripped path=w451:path)  [unwired: 1 out]
            n197 = control-ref of="Status"() -> (w452:refnum<vi>)
            n198 = call "Compile.vi"("LocalCompiledDir"=w451, "Message Box"=w452, "Compilation Type"="Compilation Type", "DevMode"=w459, "error in"=w461, "VI Path"=w460) -> ("error out"=w457:errorcluster, "Source Dir"=w458:path)  [unwired: 4 in]
            n199 = case shown="True" w459 {
              tunnel: w458 -> [w469 w473]
              tunnel: w457 -> [w470 w475]
              tunnel: w456 -> [w468 _]
              tunnel: w455 -> [w467 _]
              tunnel: [w466 w474] -> w450
              tunnel: w453 -> [w465 _]
              tunnel: w452 -> [w464 w472]
              tunnel: w451 -> [_ w471]
              tunnel: [w464 w472] -> w449
              frame False {
                n200 = call "DownloadCode.vi"("Local Version"=w468, "address"=w465, "Local Runtime"=w467, "error in"=w470, "Message Box"=w464, "Python Source"=w469) -> ("error out"=w466:errorcluster)  [unwired: 5 in]
              }
              frame True {
                n201 = call "Downloader.vi"("Message Box"=w472, "error in"=w475, "source"=w473) -> ("error out"=w477:errorcluster, "Downloader out"=w476:refnum<class "Downloader.lvclass">)  [unwired: 7 in]
                n202 = call "DownloadDevMode.vi"("LocalCompiledPath"=w471, "error in"=w477, "Downloader in"=w476) -> ("error out"=w474:errorcluster)  [unwired: 4 in, 2 out]
              }
            }
            n203 = call "Report Error.vi"("error in"=w450, "Status"=w449) -> ("error out"=w448:errorcluster)  [unwired: 9 in]
          }
          frame #2 {
            w479 = FALSE ("Running")
            n204 = Boolean To (0,1)(Boolean=w479) -> (0, 1=w480:i16)
            n205 = local write "Animated Image"(w480) -> ()
            n206 = local write "Running"(w479) -> ()
            n207 = property on="Busy" class="Ring (strict)"("Visible"=FALSE) -> ()  [unwired: 2 in, 2 out]
          }
        }
      }
    }
  }
  n208 = while "Message Generator - User Interface Event Handler" {
    tunnel: w5 -> [w483]
    stop <- w484 stop-if-true
    w485 = 200  # Event Structure Timeout (ms)
    n209 = event shown="[9] \"Compile Locally\": Value Change" {
      selector: _ -> [_ _ _ _ _ _ _ _ _ _ _ _ _]
      dyn-events: _ -> [_ _ _ _ _ _ _ _ _ _ _ _ _]
      timeout: w485 -> [_ _ _ _ _ _ _ _ _ _ _ _ _]
      tunnel: [w486 w491 _ _ _ _ _ _ _ _ _ TRUE ("Discard?") _] -> w484
      tunnel: w483 -> [w487 w489 w492 w495 w496 w498 w500 w502 w504 w506 w508 w510 w514]
      event Timeout {
        n210 = event-data() -> ()  [unwired: 2 out]
        n211 = Get Queue Status(queue=w487) -> (error out=w488:errorcluster)  [unwired: 2 in, 7 out]
        n212 = Unbundle By Name(w488) -> ("status"=w486:bool)
      }
      event Panel Close? {
        w491 = TRUE ("Discard?")
        n213 = event-data() -> ()  [unwired: 2 out]
        n214 = call "SendMessage.vi"("Name"="Exit", "message queue in"=w489) -> ()  [unwired: 5 in, 3 out]
        n215 = event-data("Discard?"=w491) -> ()  [unwired: 1 in, 1 out]
      }
      event "Open": Value Change {
        n216 = event-data() -> ()  [unwired: 2 out]
        n217 = call "SendMessage.vi"("Name"="Browse for VI", "message queue in"=w492) -> ()  [unwired: 5 in, 3 out]
      }
      event "FP": Value Change {
        n218 = event-data() -> ()  [unwired: 2 out]
        n219 = call "SendMessage.vi"("Name"="FrontPanel", "message queue in"=w495) -> ()  [unwired: 5 in, 3 out]
      }
      event "Add Ip": Value Change {
        n220 = event-data() -> ()  [unwired: 2 out]
        n221 = call "SendMessage.vi"("Name"="Add IP", "message queue in"=w496) -> ()  [unwired: 5 in, 3 out]
      }
      event "Edit IP": Value Change {
        n222 = event-data() -> ()  [unwired: 2 out]
        n223 = call "SendMessage.vi"("Name"="Edit IP", "message queue in"=w498) -> ()  [unwired: 5 in, 3 out]
      }
      event "Verify Connectivity": Value Change {
        n224 = event-data() -> ()  [unwired: 2 out]
        n225 = call "SendMessage.vi"("Name"="Verify Connectivity", "message queue in"=w500) -> ()  [unwired: 5 in, 3 out]
      }
      event "Delete IP": Value Change {
        n226 = event-data() -> ()  [unwired: 2 out]
        n227 = call "SendMessage.vi"("Name"="Delete IP", "message queue in"=w502) -> ()  [unwired: 5 in, 3 out]
      }
      event "Download": Value Change {
        n228 = event-data() -> ()  [unwired: 2 out]
        n229 = call "SendMessage.vi"("Name"="Download", "message queue in"=w504) -> ()  [unwired: 5 in, 3 out]
      }
      event "Compile Locally": Value Change {
        n230 = event-data() -> ()  [unwired: 2 out]
        n231 = call "SendMessage.vi"("Name"="Update Local", "message queue in"=w506) -> ()  [unwired: 5 in, 3 out]
      }
      event "Help": Value Change {
        n232 = event-data() -> ()  [unwired: 2 out]
        n233 = call "SendMessage.vi"("Name"="User Manual", "message queue in"=w508) -> ()  [unwired: 5 in, 3 out]
      }
      event "exit": Value Change {
        n234 = event-data() -> ()  [unwired: 2 out]
        n235 = call "SendMessage.vi"("Name"="Exit", "message queue in"=w510) -> ()  [unwired: 5 in, 3 out]
      }
      event Menu Selection (User) {
        n236 = event-data() -> ("ItemPath"=w515:string, "ItemTag"=w513:string)  [unwired: 1 out]
        n237 = call "SendMessage.vi"("Value"=w515, "Name"=w513, "message queue in"=w514) -> ()  [unwired: 4 in, 3 out]
      }
    }
  }
  n238 = while {
    tunnel: w7 -> [_]
    tunnel: w1 -> [_]
    i -> [w520]
    stop <- w522 stop-if-true
    w517 = u32 12 ("y")
    n239 = local read "Running"() -> (w519:bool)
    n240 = Quotient & Remainder(x=w520, y=w517) -> (x-y*floor(x/y)=w518:u32)  [unwired: 1 out]
    n241 = local read "StopStat"() -> (w522:bool)
    n242 = Select(t=w518, s=w519, f=w517) -> (s? t:f=→"Busy":u32)
    n243 = Wait (ms)(milliseconds to wait=u32 40) -> ()  [unwired: 1 out]
  }
  n244 = local write "StopStat"(w7) -> ()
